vi "Anritsu VNA Measure.vi"(5 "Miscellaneous Parameters":T1, 7 "Anritsu VNA":T5, 8 "error in (no error)":errorcluster, 9 "SP Stimulus":T2={"Use Instrument Settings"=FALSE, "Blank Frequencies"=FALSE, "Sweep Type"=enum."Linear", "Sweep"={"Fstart"=500.0, "Fstop"=1500.0, "Units"=enum."MHz", "Points"=201}, "Power (dBm)"=999.0, "IFBW (Hz)"=-1.0, "Sweep Time (s)"=-1.0, "Calibration"={"State"=FALSE, "String"=""}} {"Sweep Time (s)" format="%.3g"}, 10 "Parameters to Measure":T6[](array[typedef]) {"Channel" min=1 max=99 step=1; "Parameter"."Stimulus Port" min=1 step=1; "Parameter"."Response Port" min=1 step=1}, 11 "VISA Resource Name":refnum<visa-resource-name>) -> (0 "error out":errorcluster, 1 "S Parameters":cluster{"f0":dbl, "df":dbl, cdb[][]}, 2 "Parameters Measured":T6[](array[typedef]) {"Channel" min=1 max=99 step=1; "Parameter"."Stimulus Port" min=1 step=1; "Parameter"."Response Port" min=1 step=1}, 3 "dup VISA Resource Name":refnum<visa-resource-name>)   [LabVIEW 2011]
uses:
  tests/S Parameter/TypeDefs/SP Parameter to Measure.ctl
  tests/S Parameter/TypeDefs/SP Parameter.ctl
  tests/S Parameter/TypeDefs/SP Calibration State.ctl
  tests/S Parameter/TypeDefs/SP Measurement Format.ctl
  TypeDefs/Anritsu VNA Instrument Info.ctl
  tests/S Parameter/TypeDefs/SP Stimulus Parameters.ctl
  tests/S Parameter/TypeDefs/SP Frequency Units.ctl
  tests/S Parameter/TypeDefs/SP Miscellaneous Parameters.ctl
  TypeDefs/Anritsu VNA External Trigger Mode.ctl
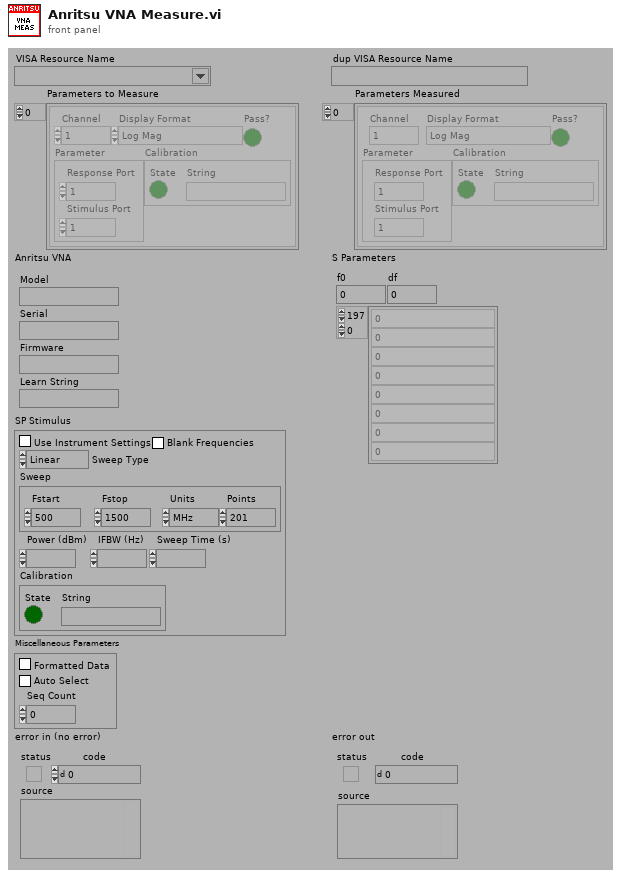
[diagram p1: front panel]
types:
  T1 = typedef "SP Miscellaneous Parameters.ctl" = cluster{"Formatted Data":bool, "Auto Select":bool, "Seq Count":u32}
  T2 = typedef "SP Stimulus Parameters.ctl" = cluster{"Use Instrument Settings":bool, "Blank Frequencies":bool, "Sweep Type":enum32{"Linear", "Logarithmic", "List", "Power", "CW"}, "Sweep":cluster{"Fstart":dbl, "Fstop":dbl, "Units":T3, "Points":i32}, "Power (dBm)":dbl, "IFBW (Hz)":dbl, "Sweep Time (s)":dbl, "Calibration":T4}
  T3 = typedef "SP Frequency Units.ctl" = enum16{"Hz", "kHz", "MHz", "GHz", "Points"}
  T4 = typedef "SP Calibration State.ctl" = cluster{"State":bool, "String":string}
  T5 = typedef "Anritsu VNA Instrument Info.ctl" = cluster{"Model":string, "Serial":string, "Firmware":string, "Learn String":string}
  T6 = typedef "SP Parameter to Measure.ctl" = cluster{"Channel":i8, "Parameter":T7, "Calibration":T4, "Display Format":T8, "Pass?":bool}
  T7 = typedef "SP Parameter.ctl" = cluster{"Stimulus Port":i8, "Response Port":i8}
  T8 = typedef "SP Measurement Format.ctl" = enum32{"Log Mag", "Phase", "Delay", "Smith (R+jX)", "Polar (Re/Im)", "Linear Mag", "SWR", "Real", "Imaginary", "Smith (Lin/Phase)", "Smith (Log/Phase)", "Smith (Real/Imag)", "Smith (G+jB)", "Polar (Lin/Phase)", "Polar (Log/Phase)", "Expanded Phase", "Positive Phase", "Inverted Smith", "Unwrapped Phase", "Power Out", "Power In", "Linear Mag/Phase", "Log Mag/Phase", "Real/Imaginary"}
  T9 = typedef "Anritsu VNA External Trigger Mode.ctl" = enum16{"Internal", "External", "Manual", "GPIB"}
  T10 = typedef "Anritsu VNA Model.ctl" = enum16{"Not Supported", "37XXXX", "MS20XXX", "MS462XX", "MS464XX"}
  T11 = typedef "Agilent VNA Measurements.ctl" = cluster{"Channel":i8, "Traces":cluster{"Trace":i8, "Parameter":T7}[]}
  T12 = typedef "Anritsu VNA Trigger Mode.ctl" = enum16{"Continuous", "Hold", "Single"}
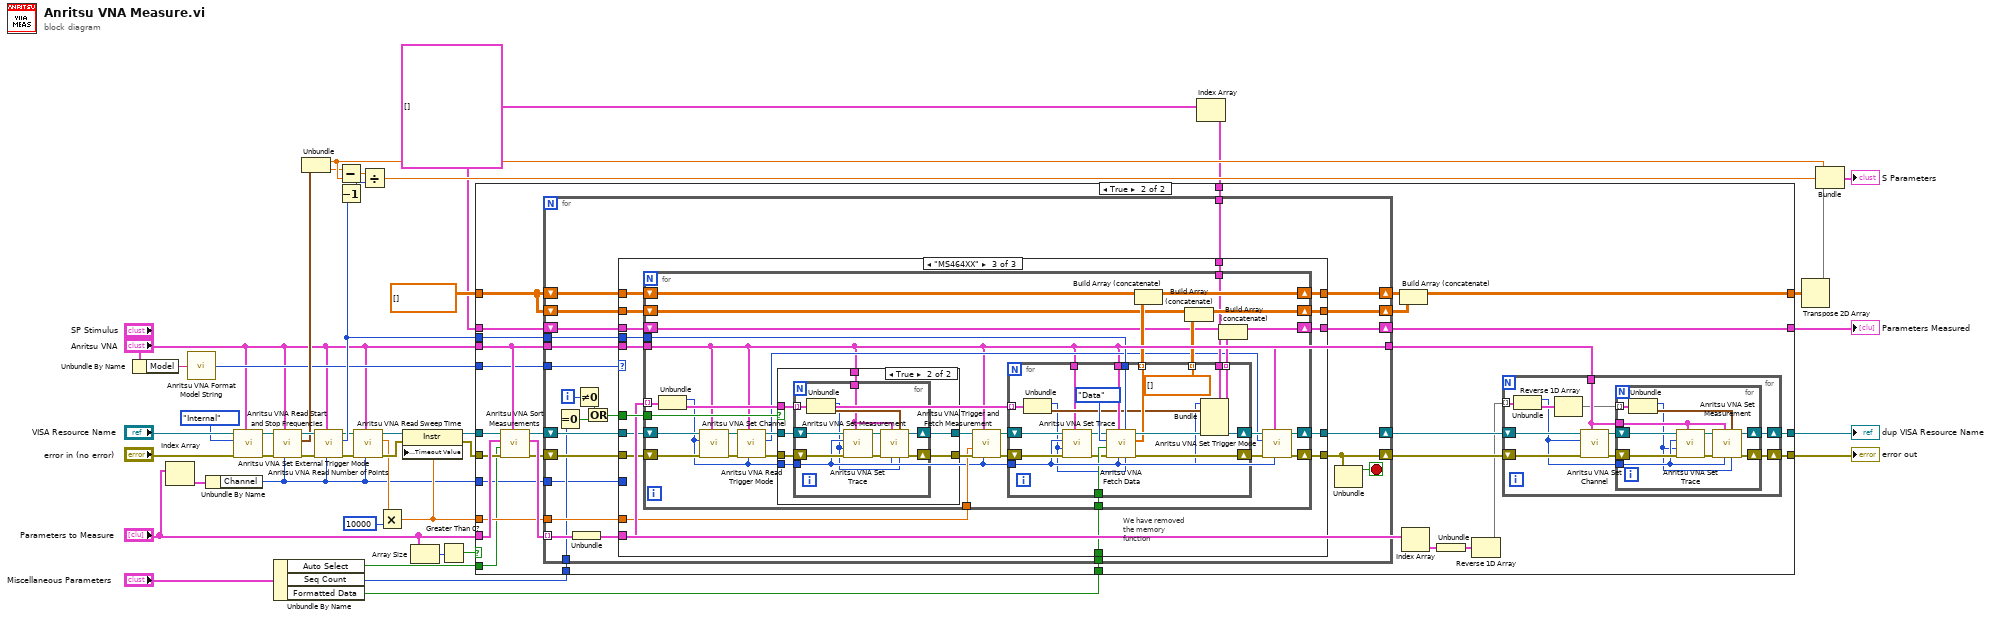
[diagram p0: block diagram]
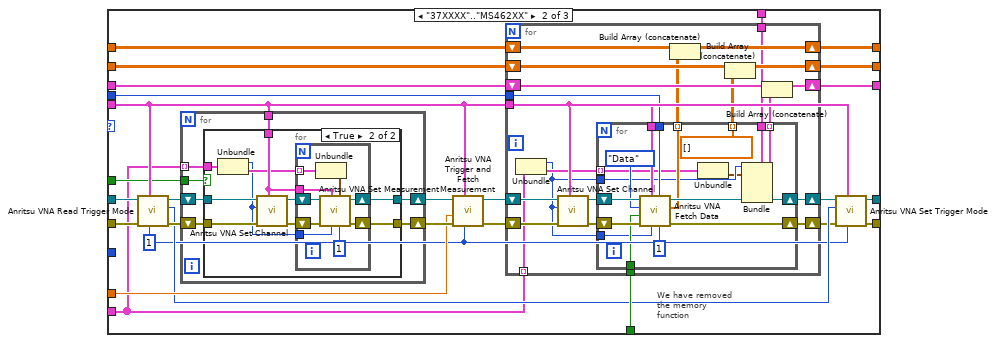
[diagram p4: hidden frame]
diagram:
  w15 = T6[] []
  n1 = Unbundle By Name("Anritsu VNA") -> ("Model"=w8:string)
  n2 = Index Array(array="Parameters to Measure") -> (element=w11:T6)  [unwired: 1 in]
  n3 = call "Anritsu VNA Format Model String.vi"("Model"=w8) -> ("Model"=w7:T10)
  n4 = Unbundle By Name(w11) -> ("Channel"=w9:i8)
  n5 = call "Anritsu VNA Set External Trigger Mode.vi"("Anritsu VNA"="Anritsu VNA", "error in (no error)"="error in (no error)", "Ext. Trigger Mode"=Anritsu_VNA_External_Trigger_Mode."Internal", "VISA Resource Name"="VISA Resource Name") -> ("error out"=w3:errorcluster, "dup VISA Resource Name"=w4:refnum<visa-resource-name>)  [unwired: 6 out]
  n6 = call "Anritsu VNA Read Start and Stop Frequencies.vi"("Channel"=w9, "Anritsu VNA"="Anritsu VNA", "error in (no error)"=w3, "VISA Resource Name"=w4) -> ("error out"=w27:errorcluster, "Start/Stop Freqs, MHz"=w13:cluster{"Fstart":dbl, "Fstop":dbl}, "dup VISA Resource Name"=w26:refnum<visa-resource-name>)  [unwired: 5 out]
  n7 = Unbundle By Name("Miscellaneous Parameters") -> ("Auto Select"=w16:bool, "Seq Count"=w12:u32, "Formatted Data"=w17:bool)
  n8 = Unbundle(w13) -> ("Fstart"=w35:dbl, "Fstop"=w34:dbl)
  n9 = call "Anritsu VNA Read Number of Points.vi"("Channel"=w9, "Anritsu VNA"="Anritsu VNA", "error in (no error)"=w27, "VISA Resource Name"=w26) -> ("error out"=w25:errorcluster, "Number Points"=w28:i32, "dup VISA Resource Name"=w24:refnum<visa-resource-name>)  [unwired: 5 out]
  n10 = Subtract(x=w34, y=w35) -> (x-y=w43:dbl)
  n11 = Decrement(x=w28) -> (x-1=w42:i32)
  n12 = call "Anritsu VNA Read Sweep Time.vi"("Channel"=w9, "Anritsu VNA"="Anritsu VNA", "error in (no error)"=w25, "VISA Resource Name"=w24) -> ("error out"=w22:errorcluster, "Sweep Time, s"=w21:dbl, "dup VISA Resource Name"=w23:refnum<visa-resource-name>)  [unwired: 5 out]
  n13 = Divide(x=w43, y=w42) -> (x/y=w40:dbl)
  n14 = Multiply(x=w21, y=u32 10000 ("Timeout (ms)")) -> (x*y=w19:dbl)
  n15 = property class="Instr"(reference=w23, error in=w22, "General Settings:Timeout Value"=w19) -> (reference out=w36:refnum<visa-resource-name>, error out=w33:errorcluster)
  n16 = Array Size(array="Parameters to Measure") -> (size(s)=w38:i32)
  n17 = Greater Than 0?(x=w38) -> (x > 0?=w37:bool)
  n18 = Index Array(array=w15) -> (element=w14:T6)  [unwired: 1 in]
  n19 = case shown="True" w37 {
    tunnel: [w48 w70] -> w30
    tunnel: w36 -> [w46 w57]
    tunnel: "Parameters to Measure" -> [_ w77]
    tunnel: [w47 w63] -> w44
    tunnel: "Anritsu VNA" -> [_ w76]
    tunnel: w33 -> [w48 w56]
    tunnel: cdb[][] [] -> [w47 w66]
    tunnel: [w46 w69] -> w29
    tunnel: w17 -> [_ w62]
    tunnel: [w45 w61] -> w31
    tunnel: w15 -> [w45 w60]
    tunnel: w19 -> [_ w59]
    tunnel: w28 -> [_ w58]
    tunnel: w16 -> [_ w53]
    tunnel: w14 -> [_ w52]
    tunnel: w12 -> [_ w51]
    tunnel: w9 -> [_ w50]
    tunnel: w7 -> [_ w49]
    frame False {
    }
    frame True {
      n20 = call "Anritsu VNA Sort Measurements.vi"("Anritsu VNA"=w76, "error in (no error)"=w56, "Auto Select"=w53, "Parameters to Measure"=w77, "VISA Resource Name"=w57) -> ("error out"=w54:errorcluster, "Sorted Measurements"=w75:cluster{"Measurements":T11[]}[], "dup VISA Resource Name"=w55:refnum<visa-resource-name>)  [unwired: 4 out]
      n21 = for {
        shift-right: [w97] -> w71
        shift-left: w54 -> [w98]
        tunnel: w75 -> [w102] mode=indexing
        tunnel: w76 -> [w87]
        shift-right: [w90] -> w64
        shift-left: w66 -> [w94]
        shift-right: [w96] -> w72
        shift-left: w55 -> [w99]
        tunnel: [w87] -> w67
        shift-right: [w89] -> w65
        shift-left: w66 -> [w93]
        tunnel: w62 -> [w101]
        shift-right: [w91] -> w61
        shift-left: w60 -> [w92]
        tunnel: w59 -> [w100]
        tunnel: w58 -> [w88]
        tunnel: w52 -> [w85]
        tunnel: w51 -> [w81]
        tunnel: w50 -> [w79]
        tunnel: w49 -> [w78]
        i -> [w82]
        stop <- w95 stop-if-true
        n22 = Equal To 0?(x=w81) -> (x = 0?=w83:bool)
        n23 = Unbundle(w102) -> ("Measurements"=w86:T11[])
        n24 = Not Equal To 0?(x=w82) -> (x != 0?=w84:bool)
        n25 = Or(x=w84, y=w83) -> (x .or. y?=w80:bool)
        n26 = case shown="\"MS464XX\"" w78 {
          tunnel: w101 -> [_ w132 w204]
          tunnel: w100 -> [_ w129 w214]
          tunnel: w99 -> [w104 w128 w215]
          tunnel: w98 -> [w103 w127 w216]
          tunnel: [w103 w121 w209] -> w97
          tunnel: [w104 w120 w208] -> w96
          tunnel: w94 -> [w107 w119 w205]
          tunnel: w93 -> [w106 w118 w212]
          tunnel: w92 -> [w105 w117 w207]
          tunnel: [w105 w116 w202] -> w91
          tunnel: [w107 w115 w203] -> w90
          tunnel: [w106 w114 w206] -> w89
          tunnel: w88 -> [_ w113 w211]
          tunnel: w87 -> [_ w112 w213]
          tunnel: w86 -> [_ w109 w217]
          tunnel: w85 -> [_ w111 w210]
          tunnel: w80 -> [_ w110 w218]
          tunnel: w79 -> [_ _ _]
          frame "Not Supported" {
          }
          frame "37XXXX".."MS462XX" {
            w108 = i8 1 ("Channel")
            # "We have removed\nthe memory\nfunction"
            n27 = call "Anritsu VNA Read Trigger Mode.vi"("Channel"=w108, "Anritsu VNA"=w112, "error in (no error)"=w127, "VISA Resource Name"=w128) -> ("error out"=w125:errorcluster, "Trigger Mode"=w124:T12, "dup VISA Resource Name"=w126:refnum<visa-resource-name>)  [unwired: 5 out]
            n28 = for {
              tunnel: w112 -> [w177]
              tunnel: w109 -> [w178] mode=indexing
              shift-right: [w179] -> w131
              shift-left: w125 -> [w175]
              shift-right: [w180] -> w130
              shift-left: w126 -> [w176]
              tunnel: w110 -> [w174]
              n29 = case shown="True" w174 {
                tunnel: [w182 w192] -> w180
                tunnel: [w181 w191] -> w179
                tunnel: w178 -> [_ w190]
                tunnel: w177 -> [_ w187]
                tunnel: w176 -> [w182 w186]
                tunnel: w175 -> [w181 w185]
                frame False {
                  # "Save time because we know that\nthe previous run set these\nmeasurements back to the first\nparameters.  The cannot be skipped\nif it is the second measurement in a\nrun though or if it is the first time\nthrough."
                }
                frame True {
                  n30 = Unbundle(w190) -> ("Channel"=w183:i8, "Traces"=w184:cluster{"Trace":i8, "Parameter":T7}[])
                  n31 = call "Anritsu VNA Set Channel.vi"("Anritsu VNA"=w187, "error in (no error)"=w185, "Channel"=w183, "VISA Resource Name"=w186) -> ("error out"=w188:errorcluster, "dup VISA Resource Name"=w189:refnum<visa-resource-name>)  [unwired: 6 out]
                  n32 = for {
                    tunnel: w187 -> [w197]
                    shift-right: [w201] -> w192
                    shift-left: w189 -> [w196]
                    shift-right: [w200] -> w191
                    shift-left: w188 -> [w195]
                    tunnel: w184 -> [w199] mode=indexing
                    tunnel: w183 -> [w194]
                    n33 = Unbundle(w199) -> ("Parameter"=w198:T7)  [unwired: 1 out]
                    n34 = call "Anritsu VNA Set Measurement.vi"("Trace"=i8 1, "Parameter"=w198, "Channel"=w194, "Anritsu VNA"=w197, "error in (no error)"=w195, "VISA Resource Name"=w196) -> ("error out"=w200:errorcluster, "dup VISA Resource Name"=w201:refnum<visa-resource-name>)  [unwired: 1 in, 3 out]
                  }
                }
              }
            }
            n35 = call "Anritsu VNA Trigger and Fetch Measurement.vi"("Channel"=w108, "Anritsu VNA"=w112, "error in (no error)"=w131, "Timeout, ms (10000)"=w129, "VISA Resource Name"=w130) -> ("error out"=w134:errorcluster, "dup VISA Resource Name"=w133:refnum<visa-resource-name>)  [unwired: 1 in, 4 out]
            n36 = for {
              shift-right: [w150] -> w122
              shift-left: w134 -> [w156]
              shift-right: [w151] -> w123
              shift-left: w133 -> [w153]
              tunnel: w132 -> [w152]
              shift-right: [w144] -> w115
              shift-left: w119 -> [w149]
              shift-right: [w145] -> w114
              shift-left: w118 -> [w148]
              shift-right: [w146] -> w116
              shift-left: w117 -> [w147]
              tunnel: w113 -> [w142]
              tunnel: w112 -> [w141]
              tunnel: w109 -> [w140] mode=indexing
              tunnel: w111 -> [w138]
              n37 = Unbundle(w140) -> ("Channel"=w135:i8, "Traces"=w137:cluster{"Trace":i8, "Parameter":T7}[])
              n38 = call "Anritsu VNA Set Channel.vi"("Anritsu VNA"=w141, "error in (no error)"=w156, "Channel"=w135, "VISA Resource Name"=w153) -> ("error out"=w155:errorcluster, "dup VISA Resource Name"=w154:refnum<visa-resource-name>)  [unwired: 6 out]
              n39 = for {
                tunnel: w152 -> [w170]
                tunnel: [w167] -> w143 mode=indexing
                tunnel: w142 -> [w166]
                tunnel: w141 -> [w165]
                shift-right: [w169] -> w151
                shift-left: w154 -> [w172]
                shift-right: [w168] -> w150
                shift-left: w155 -> [w173]
                tunnel: [cdb[] [] ("Data (real+imag)")] -> w139 mode=indexing
                tunnel: w138 -> [w163]
                tunnel: w135 -> [w162]
                tunnel: w137 -> [w161] mode=indexing
                tunnel: [w159] -> w136 mode=indexing
                tunnel: w135 -> [w158]
                n40 = call "Anritsu VNA Fetch Data.vi"("Trace"=i8 1, "Number of Points"=w166, "Channel"=w158, "Anritsu VNA"=w165, "error in (no error)"=w173, "Formatted Data?"=w170, "Data to Read (Data)"=enum16{"Data", "Memory"}."Data", "VISA Resource Name"=w172) -> ("error out"=w168:errorcluster, "Data (real+imag)"=w167:cdb[], "dup VISA Resource Name"=w169:refnum<visa-resource-name>)  [unwired: 1 out]
                n41 = Unbundle(w161) -> ("Parameter"=w160:T7)  [unwired: 1 out]
                n42 = Bundle(cluster=w163, "Channel"=w162, "Parameter"=w160) -> (w159:T6)  [unwired: 3 out]
              }
              n43 = Build Array (concatenate)(w149, w143) -> (w144:cdb[][])
              n44 = Build Array (concatenate)(w148, w139) -> (w145:cdb[][])
              n45 = Build Array (concatenate)(w147, w136) -> (w146:T6[])
            }
            n46 = call "Anritsu VNA Set Trigger Mode.vi"("Channel"=w108, "Anritsu VNA"=w112, "error in (no error)"=w122, "Trigger Mode"=w124, "VISA Resource Name"=w123) -> ("error out"=w121:errorcluster, "dup VISA Resource Name"=w120:refnum<visa-resource-name>)  [unwired: 5 out]
          }
          frame "MS464XX" {
            # "We have removed\nthe memory\nfunction"
            n47 = for {
              tunnel: w217 -> [w248] mode=indexing
              shift-right: [w222] -> w209
              shift-left: w216 -> [w250]
              shift-right: [w223] -> w208
              shift-left: w215 -> [w249]
              tunnel: w218 -> [w251]
              tunnel: w214 -> [w241]
              tunnel: w213 -> [w219]
              shift-right: [w232] -> w203
              shift-left: w205 -> [w235]
              shift-right: [w231] -> w206
              shift-left: w212 -> [w234]
              shift-right: [w230] -> w202
              shift-left: w207 -> [w233]
              tunnel: w211 -> [w228]
              tunnel: w210 -> [w227]
              tunnel: w204 -> [w226]
              n48 = Unbundle(w248) -> ("Channel"=w221:i8, "Traces"=w229:cluster{"Trace":i8, "Parameter":T7}[])
              n49 = call "Anritsu VNA Set Channel.vi"("Anritsu VNA"=w219, "error in (no error)"=w250, "Channel"=w221, "VISA Resource Name"=w249) -> ("error out"=w247:errorcluster, "dup VISA Resource Name"=w244:refnum<visa-resource-name>)  [unwired: 6 out]
              n50 = call "Anritsu VNA Read Trigger Mode.vi"("Channel"=w221, "Anritsu VNA"=w219, "error in (no error)"=w247, "VISA Resource Name"=w244) -> ("error out"=w246:errorcluster, "Trigger Mode"=w220:T12, "dup VISA Resource Name"=w245:refnum<visa-resource-name>)  [unwired: 5 out]
              n51 = case shown="True" w251 {
                tunnel: [w272 w279] -> w243
                tunnel: [w271 w278] -> w242
                tunnel: w245 -> [w272 w276]
                tunnel: w246 -> [w271 w275]
                tunnel: w229 -> [_ w277]
                tunnel: w221 -> [_ w274]
                tunnel: w219 -> [_ w273]
                frame False {
                  # "Save time because we know that\nthe previous run set these\nmeasurements back to the first\nparameters.  The cannot be skipped\nif it is the second measurement in a\nrun though or if it is the first time\nthrough."
                }
                frame True {
                  n52 = for {
                    shift-right: [w290] -> w279
                    shift-left: w276 -> [w285]
                    shift-right: [w289] -> w278
                    shift-left: w275 -> [w286]
                    tunnel: w277 -> [w288] mode=indexing
                    tunnel: w274 -> [w282]
                    tunnel: w273 -> [w280]
                    n53 = Unbundle(w288) -> ("Trace"=w281:i8, "Parameter"=w287:T7)
                    n54 = call "Anritsu VNA Set Trace.vi"("Anritsu VNA"=w280, "error in (no error)"=w286, "Trace"=w281, "Channel"=w282, "VISA Resource Name"=w285) -> ("error out"=w283:errorcluster, "dup VISA Resource Name"=w284:refnum<visa-resource-name>)  [unwired: 5 out]
                    n55 = call "Anritsu VNA Set Measurement.vi"("Trace"=w281, "Parameter"=w287, "Channel"=w282, "Anritsu VNA"=w280, "error in (no error)"=w283, "VISA Resource Name"=w284) -> ("error out"=w289:errorcluster, "dup VISA Resource Name"=w290:refnum<visa-resource-name>)  [unwired: 1 in, 3 out]
                  }
                }
              }
              n56 = call "Anritsu VNA Trigger and Fetch Measurement.vi"("Channel"=w221, "Anritsu VNA"=w219, "error in (no error)"=w242, "Timeout, ms (10000)"=w241, "VISA Resource Name"=w243) -> ("error out"=w236:errorcluster, "dup VISA Resource Name"=w237:refnum<visa-resource-name>)  [unwired: 1 in, 4 out]
              n57 = for {
                tunnel: w226 -> [w269]
                tunnel: [w266] -> w238 mode=indexing
                tunnel: w228 -> [w265]
                tunnel: w219 -> [w264]
                shift-right: [w268] -> w224
                shift-left: w237 -> [w255]
                shift-right: [w267] -> w225
                shift-left: w236 -> [w258]
                tunnel: [cdb[] [] ("Data (real+imag)")] -> w239 mode=indexing
                tunnel: w227 -> [w262]
                tunnel: w229 -> [w261] mode=indexing
                tunnel: [w259] -> w240 mode=indexing
                tunnel: w221 -> [w254]
                tunnel: w219 -> [w252]
                n58 = Unbundle(w261) -> ("Trace"=w253:i8, "Parameter"=w260:T7)
                n59 = call "Anritsu VNA Set Trace.vi"("Anritsu VNA"=w252, "error in (no error)"=w258, "Trace"=w253, "Channel"=w254, "VISA Resource Name"=w255) -> ("error out"=w257:errorcluster, "dup VISA Resource Name"=w256:refnum<visa-resource-name>)  [unwired: 5 out]
                n60 = call "Anritsu VNA Fetch Data.vi"("Trace"=w253, "Number of Points"=w265, "Channel"=w254, "Anritsu VNA"=w264, "error in (no error)"=w257, "Formatted Data?"=w269, "Data to Read (Data)"=enum16{"Data", "Memory"}."Data", "VISA Resource Name"=w256) -> ("error out"=w267:errorcluster, "Data (real+imag)"=w266:cdb[], "dup VISA Resource Name"=w268:refnum<visa-resource-name>)  [unwired: 1 out]
                n61 = Bundle(cluster=w262, "Channel"=w254, "Parameter"=w260) -> (w259:T6)  [unwired: 3 out]
              }
              n62 = Build Array (concatenate)(w235, w238) -> (w232:cdb[][])
              n63 = Build Array (concatenate)(w234, w239) -> (w231:cdb[][])
              n64 = Build Array (concatenate)(w233, w240) -> (w230:T6[])
              n65 = call "Anritsu VNA Set Trigger Mode.vi"("Channel"=w221, "Anritsu VNA"=w219, "error in (no error)"=w225, "Trigger Mode"=w220, "VISA Resource Name"=w224) -> ("error out"=w222:errorcluster, "dup VISA Resource Name"=w223:refnum<visa-resource-name>)  [unwired: 5 out]
            }
          }
        }
        n66 = Unbundle(w97) -> ("status"=w95:bool)  [unwired: 2 out]
      }
      n67 = Build Array (concatenate)(w64, w65) -> (w63:cdb[][])
      n68 = Index Array(array=w75) -> (element=w74:cluster{"Measurements":T11[]})  [unwired: 1 in]
      n69 = Unbundle(w74) -> ("Measurements"=w73:T11[])
      n70 = Reverse 1D Array(array=w73) -> (reversed array=w68:T11[])
      n71 = for {
        tunnel: w67 -> [w298]
        tunnel: w68 -> [w299] mode=indexing
        shift-right: [w300] -> w70
        shift-left: w71 -> [w297]
        shift-right: [w301] -> w69
        shift-left: w72 -> [w296]
        n72 = Unbundle(w299) -> ("Channel"=w291:i8, "Traces"=w293:cluster{"Trace":i8, "Parameter":T7}[])
        n73 = Reverse 1D Array(array=w293) -> (reversed array=w292:cluster{"Trace":i8, "Parameter":T7}[])
        n74 = call "Anritsu VNA Set Channel.vi"("Anritsu VNA"=w298, "error in (no error)"=w297, "Channel"=w291, "VISA Resource Name"=w296) -> ("error out"=w295:errorcluster, "dup VISA Resource Name"=w294:refnum<visa-resource-name>)  [unwired: 6 out]
        n75 = for {
          tunnel: w298 -> [w304]
          shift-right: [w312] -> w301
          shift-left: w294 -> [w307]
          shift-right: [w311] -> w300
          shift-left: w295 -> [w308]
          tunnel: w292 -> [w310] mode=indexing
          tunnel: w291 -> [w303]
          n76 = Unbundle(w310) -> ("Trace"=w302:i8, "Parameter"=w309:T7)
          n77 = call "Anritsu VNA Set Trace.vi"("Anritsu VNA"=w304, "error in (no error)"=w308, "Trace"=w302, "Channel"=w303, "VISA Resource Name"=w307) -> ("error out"=w305:errorcluster, "dup VISA Resource Name"=w306:refnum<visa-resource-name>)  [unwired: 5 out]
          n78 = call "Anritsu VNA Set Measurement.vi"("Trace"=w302, "Parameter"=w309, "Channel"=w303, "Anritsu VNA"=w304, "error in (no error)"=w305, "VISA Resource Name"=w306) -> ("error out"=w311:errorcluster, "dup VISA Resource Name"=w312:refnum<visa-resource-name>)  [unwired: 1 in, 3 out]
        }
      }
    }
  }
  "error out" <- w30
  "Parameters Measured" <- w31
  "dup VISA Resource Name" <- w29
  n79 = Transpose 2D Array(2D array=w44) -> (transposed array=w39:cdb[][])
  n80 = Bundle("Fstart"=w35, w40, w39) -> (→"S Parameters":cluster{"Fstart":dbl, dbl, cdb[][]})  [unwired: 1 out]
